vi "ROI Point1.vi"(11 "ROI":T1) -> (2 "y":i32, 3 "x":i32)   [LabVIEW 2015]
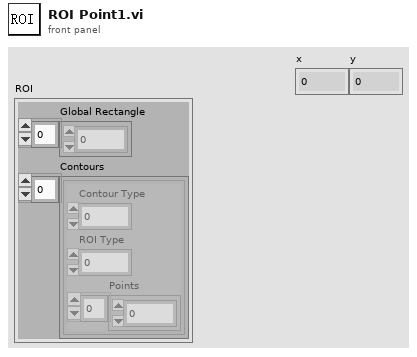
[diagram p1: front panel]
types:
  T1 = cluster{"Global Rectangle":i32[], "Contours":cluster{"Contour Type":u32, "ROI Type":u32, "Points":i32[]}[]}
  T2 = cluster{"Contour Type":u32, "ROI Type":u32, "Points":i32[]}[]
  T3 = cluster{"Contour Type":u32, "ROI Type":u32, "Points":i32[]}
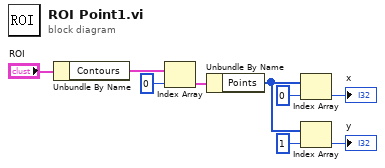
[diagram p0: block diagram]
diagram:
  n1 = Unbundle By Name("ROI") -> ("Contours"=w9:T2)
  n2 = Index Array(array=w9, index=0) -> (element=w6:T3)
  n3 = Unbundle By Name(w6) -> ("Points"=w3:i32[])
  n4 = Index Array(array=w3, index=0) -> (element=→"x":i32)
  n5 = Index Array(array=w3, index=1) -> (element=→"y":i32)
